vi "LOGIC_GetNextImage.vi"(11 "DBS Ref":T1) -> (1 "raw bpp":i32, 2 "next image info":T2={"name"="/home/bonati/images/mono051", "number"=51, "bpp"=32, "write "=TRUE, "imageToRead"=1, "rootName"="/home/bonati/images/mono"})   [LabVIEW 2016]
uses:
  DBSHAND/private/vis/DatabaseHand_RefNum.ctl
  Common/public/vis/CMN_FVAR_action.ctl
  DBSHAND/private/vis/DatabaseHand_Element_Get(string).vi
  DBSHAND/private/vis/DatabaseHand_Element_Get(bool).vi
  DBSHAND/private/vis/DatabaseHand_Element_Get(I32).vi
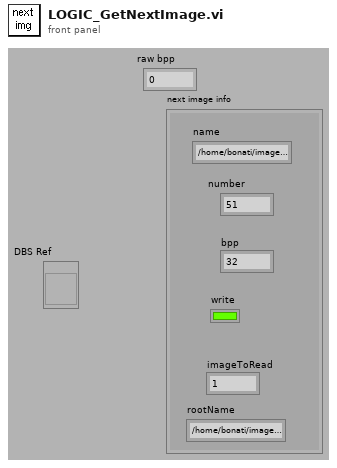
[diagram p1: front panel]
types:
  T1 = typedef "DatabaseHand_RefNum.ctl" = refnum<vi>
  T2 = cluster{"name":string, "number":i32, "bpp":u8, "write ":bool, "imageToRead":u16, "rootName":string}
  T3 = typedef "CMN_FVAR_action.ctl" = enum16{"read", "write"}
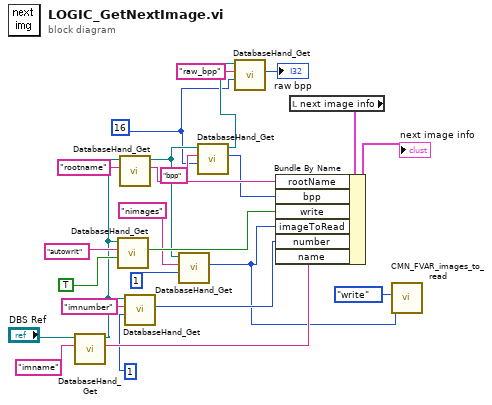
[diagram p0: block diagram]
diagram:
  w2 = 16
  n1 = call-poly "DatabaseHand_Get.vi"("name"="imname", "Database RefNum in"="DBS Ref") -> ("value"=w21:string, "Database RefNum out"=w14:T1)  [unwired: 3 in, 5 out]
  n2 = call-poly "DatabaseHand_Get.vi"("default value"=TRUE, "name"="autowrit", "Database RefNum in"=w14) -> ("value"=w18:bool)  [unwired: 2 in, 6 out]
  n3 = call-poly "DatabaseHand_Get.vi"("name"="rootname", "Database RefNum in"=w14) -> ("value"=w12:string, "Database RefNum out"=w7:T1)  [unwired: 3 in, 5 out]
  n4 = call-poly "DatabaseHand_Get.vi"("default value"=1 ("ImageNumber"), "name"="imnumber", "Database RefNum in"=w14) -> ("value"=w15:i32)  [unwired: 2 in, 6 out]
  n5 = call-poly "DatabaseHand_Get.vi"("default value"=1 ("ImageNumber"), "name"="nimages", "Database RefNum in"=w7) -> ("value"=w8:i32)  [unwired: 2 in, 6 out]
  n6 = call-poly "DatabaseHand_Get.vi"("default value"=w2, "name"="bpp", "Database RefNum in"=w7) -> ("value"=w5:i32, "Database RefNum out"=w4:T1)  [unwired: 2 in, 5 out]
  n7 = call-poly "DatabaseHand_Get.vi"("default value"=w2, "name"="raw_bpp", "Database RefNum in"=w4) -> ("value"=→"raw bpp":i32)  [unwired: 2 in, 6 out]
  n8 = local read "next image info"() -> (w25:T2)
  n9 = Bundle By Name(cluster=w25, "rootName"=w12, "bpp"=w5, "write"=w18, "imageToRead"=w8, "number"=w15, "name"=w21) -> (→"next image info":T2)
  n10 = call "CMN_FVAR_images_to_read.vi"("value in"=w8, "action"=CMN_FVAR_action."write") -> ()  [unwired: 9 out]
